vi "Send.vi"(5 "Record Topic Name?":bool, 7 "Message Priority":T1, 8 "error in (no error)":errorcluster, 9 "Timeout":i32, 10 "Message":refnum<class "Message Interface.lvclass">, 11 "Message Transport Notifier in":refnum<class "Message Transport Notifier.lvclass">) -> (0 "error out":errorcluster, 2 "Timed Out?":bool, 3 "Message Transport Notifier out":refnum<class "Message Transport Notifier.lvclass">)   [LabVIEW 2016, in "Stream Mediator.lvlib" / "Message Transport Notifier.lvclass"]
doc: "--\nCopyright © 2017 Composed SystemsI All rights reserved.\n\nAuthor: Jon McBee <jon.mcbee@composed.io>\n\nThis library is provided \"AS IS\" ,WITHOUT WARRANTIES OR\nCONDITIONS OF ANY KIND, either express or implied.\n\nComposed Systems -- composed.io\n\nStream 0.0.1.1\nJon McBee - Composed Systems\nCopyright (c) 2017, Composed Systems"
uses:
  <userlib>/Composed Systems/Stream/Mediator/Classes/Message Transport Notifier/Message Transport Notifier.lvclass
  C:/Program Files (x86)/National Instruments/LabVIEW 2016/user.lib/Composed Systems/Stream/Mediator/Classes/Message Transport Interface/Message Transport Interface.lvclass
  <userlib>/Composed Systems/Stream/Mediator/Classes/Message Interface/Message Interface.lvclass
  <userlib>/Composed Systems/Stream/Mediator/Classes/Message Transport Interface/Message Priority.ctl
  <userlib>/Composed Systems/Stream/Mediator/Classes/Message Interface/Message Interface.lvclass/Message Interface.ctl
  <userlib>/Composed Systems/Stream/Mediator/Classes/Message Transport Notifier/Message Transport Notifier.lvclass/Message Transport Notifier.ctl
  <userlib>/Composed Systems/Stream/Mediator/Classes/Message Transport Interface/Message Transport Interface.lvclass
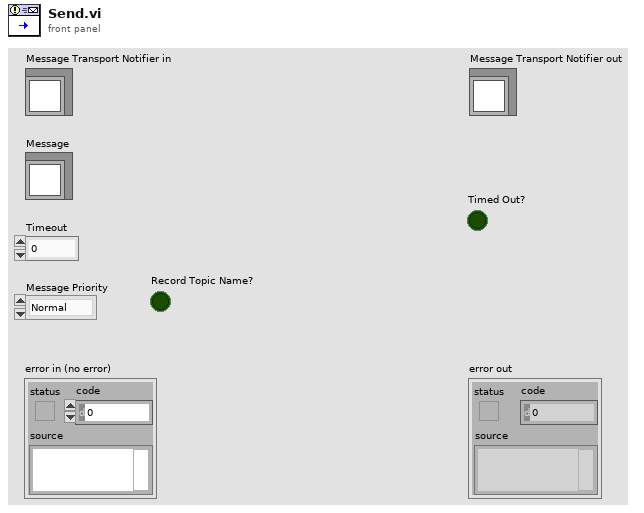
[diagram p1: front panel]
types:
  T1 = typedef "Stream Mediator.lvlib/Message Transport Interface.lvclass/Message Priority.ctl" = enum16{"Normal", "High"}
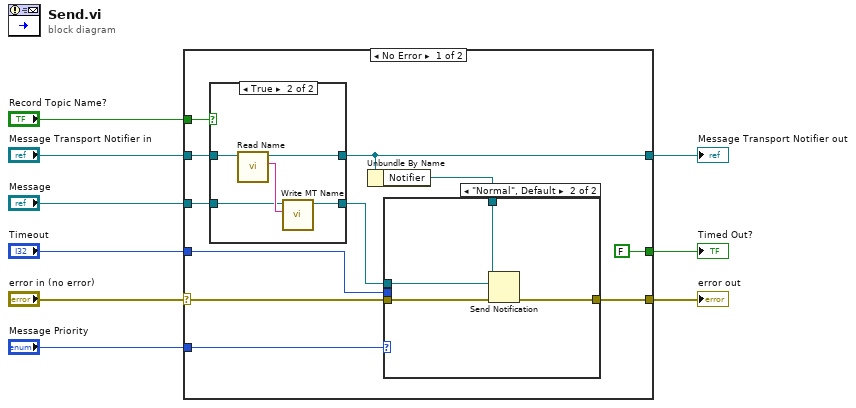
[diagram p0: block diagram]
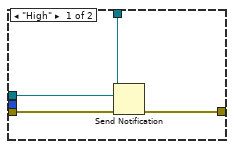
[diagram p3: hidden frame]
diagram:
  n1 = case shown="No Error" "error in (no error)" {
    selector: "error in (no error)" -> [w19 w36]
    tunnel: [w18 w36] -> w8
    tunnel: "Message Priority" -> [w20 _]
    tunnel: "Timeout" -> [w16 _]
    tunnel: "Message" -> [w12 _]
    tunnel: "Message Transport Notifier in" -> [w14 w37]
    tunnel: [w13 w37] -> w3
    tunnel: [FALSE _] -> w2
    tunnel: "Record Topic Name?" -> [w10 _]
    frame No Error {
      n2 = case shown="True" w10 {
        tunnel: w14 -> [w22 w26]
        tunnel: [w22 w25] -> w13
        tunnel: w12 -> [w21 w24]
        tunnel: [w21 w23] -> w11
        frame False {
        }
        frame True {
          n3 = call <userlib>:"Read Name.vi"("Message Transport Interface in"=w26) -> ("Name"=w27:string, "Message Transport Interface out"=w25:refnum<class "Message Transport Notifier.lvclass">)  [unwired: 8 in, 1 out]
          n4 = call <userlib>:"Write MT Name.vi"("MT Name"=w27, "Message Interface in"=w24) -> ("Message Interface out"=w23:refnum<class "Message Interface.lvclass">)  [unwired: 9 in]
        }
      }
      n5 = Unbundle By Name(w13) -> ("Notifier"=w17:refnum<notifier>)
      n6 = case shown="\"Normal\", Default" w20 {
        tunnel: [w29 w33] -> w18
        tunnel: w19 -> [w30 w34]
        tunnel: w17 -> [w31 w35]
        tunnel: w11 -> [w28 w32]
        tunnel: w16 -> [_ _]
        frame "High" {
          n7 = Send Notification(notification=w28, notifier=w31, error in (no error)=w30) -> (error out=w29:errorcluster)  [unwired: 1 out]
        }
        frame "Normal", Default {
          n8 = Send Notification(notification=w32, notifier=w35, error in (no error)=w34) -> (error out=w33:errorcluster)  [unwired: 1 out]
        }
      }
    }
    frame Error {
    }
  }
  "error out" <- w8
  "Message Transport Notifier out" <- w3
  "Timed Out?" <- w2
